vi "ODE Solver formula string.vi"(7 "ODE RHS":T1, 8 "error in (no error)":errorcluster, 10 "simulation parameters":T2={"Initial Time"=0.0, "Final Time"=10.0, "Time Step"=0.1, "Absolute Tolerance"=0.001, "Relative Tolerance"=0.001, "Continuous Solver"=enum."Runge-Kutta 45 (variable)", "Discrete Time Step"=1.0, "Minimum Time Step"=1e-08, "Maximum Time Step"=1.0, "Initial Time Step"=0.01} {"Initial Time Step" min=0.0; "Maximum Time Step" min=0.0}, 11 "x0":dbl[](array[numeric])) -> (0 "error out":errorcluster, 2 "outputs":dbl[][](array[numeric]), 3 "times":dbl[](array[numeric]))   [LabVIEW 2010, in "NI_Gmath.lvlib"]
doc: "Solves ordinary differential equations with initial conditions of the following form: X'=F(X,t). You must manually select the polymorphic instance to use."
uses:
  NI_Gmath.lvlib
  SIM Diagram Parameters.ctl
  SIM Continuous Solvers.ctl
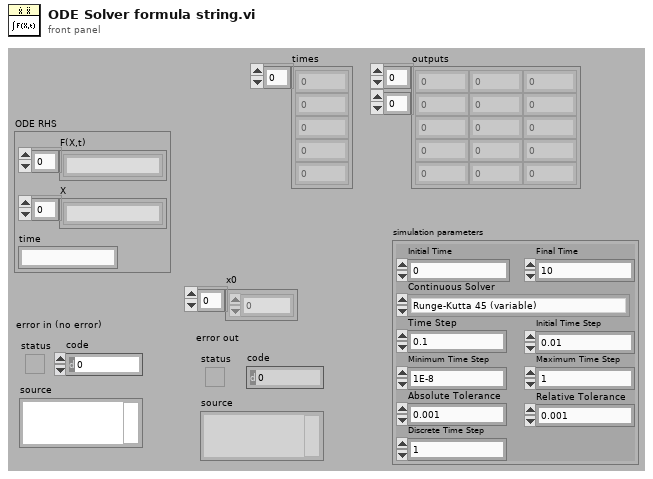
[diagram p1: front panel]
types:
  T1 = cluster{"F(X,t)":string[], "X":string[], "time":string}
  T2 = typedef "SIM Diagram Parameters.ctl" = cluster{"Initial Time":dbl, "Final Time":dbl, "Time Step":dbl, "Absolute Tolerance":dbl, "Relative Tolerance":dbl, "Continuous Solver":T3, "Discrete Time Step":dbl, "Minimum Time Step":dbl, "Maximum Time Step":dbl, "Initial Time Step":dbl}
  T3 = typedef "SIM Continuous Solvers.ctl" = enum16{"Runge-Kutta 1 (Euler)", "Runge-Kutta 2", "Runge-Kutta 3", "Runge-Kutta 4", "Runge-Kutta 23 (variable)", "Runge-Kutta 45 (variable)", "BDF (variable)", "Adams-Moulton (variable)", "Rosenbrock (variable)", "Discrete States Only"}
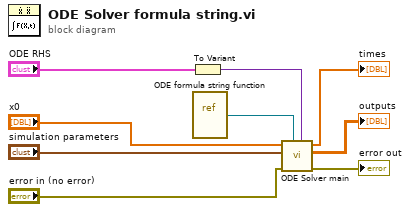
[diagram p0: block diagram]
diagram:
  n1 = To Variant(anything="ODE RHS") -> (Variant=w7:variant)
  n2 = vi-ref "ODE formula string function.vi"() -> ("vi reference"=w9:refnum<vi>)
  n3 = call "ODE Solver main.vi"("data"=w7, "ODE F(X,t)"=w9, "error in (no error)"="error in (no error)", "simulation parameters"="simulation parameters", "x0"="x0") -> ("error out"=→"error out":errorcluster, "outputs"=→"outputs":dbl[][], "times"=→"times":dbl[])  [unwired: 4 in]
